vi "MapaIntensidade-FROG.vi"() -> ()   [LabVIEW 2014]
doc: "Mapa de Intensidade FROG\n\nAndré Romero - 2022\nandretec@ifsc.usp.br"
uses:
  FROG-GlobalVar.vi
  <vilib>/Utility/file.llb/Write To Spreadsheet File (DBL).vi
panel:
  in  "stop":bool
  out "Intensity Graph":dbl[][](graph)
  out "Numeric 2":i32
  out "Numeric":i32=4
  out "appended array":dbl[](array[numeric])
  out "Progresso":i32=4
  out "size(s) 2":i32[](array[numeric])=[5, 5]
  out "Array":dbl[][](array[numeric])=[[222.8, 222.8, 222.8, 221.0, 0.0], [220.2, 220.7, 221.6, 222.2, 222.3], [222.4, 222.4, 222.4, 222.5, 0.0], [222.5, 222.5, 222.5, 222.5, 222.5], [0.0, 0.0, 0.0, 0.0, 0.0]]
  out "GO":bool
  out "Temporal FWHM":dbl
  in  "milliseconds to wait":u32=1500
  out "size(s)":i32
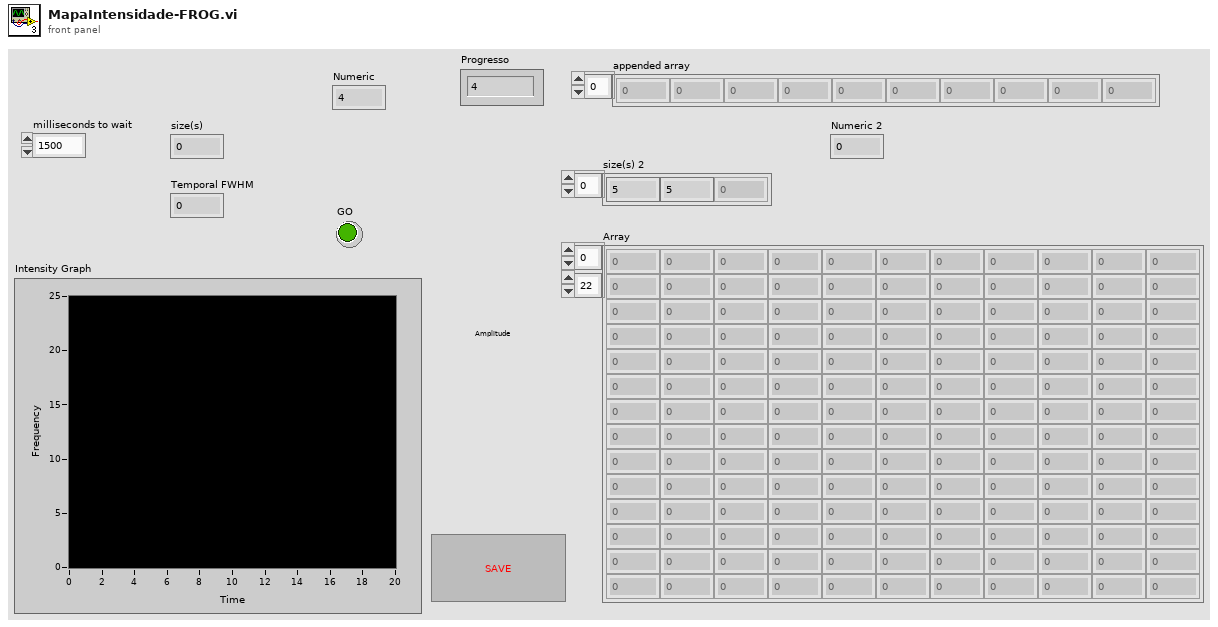
[diagram p1: front panel]
types:
  T1 = typedef "FROG.ctl" = cluster{"Delay increment":dbl, "Center Wavelength":dbl, "Frog Error was":dbl, "Temporal FWHM":dbl, "Spectral FWHM":dbl, "FWHM Time-Bandwidth Product":dbl, "RMS Time-Bandwidth Product":dbl}
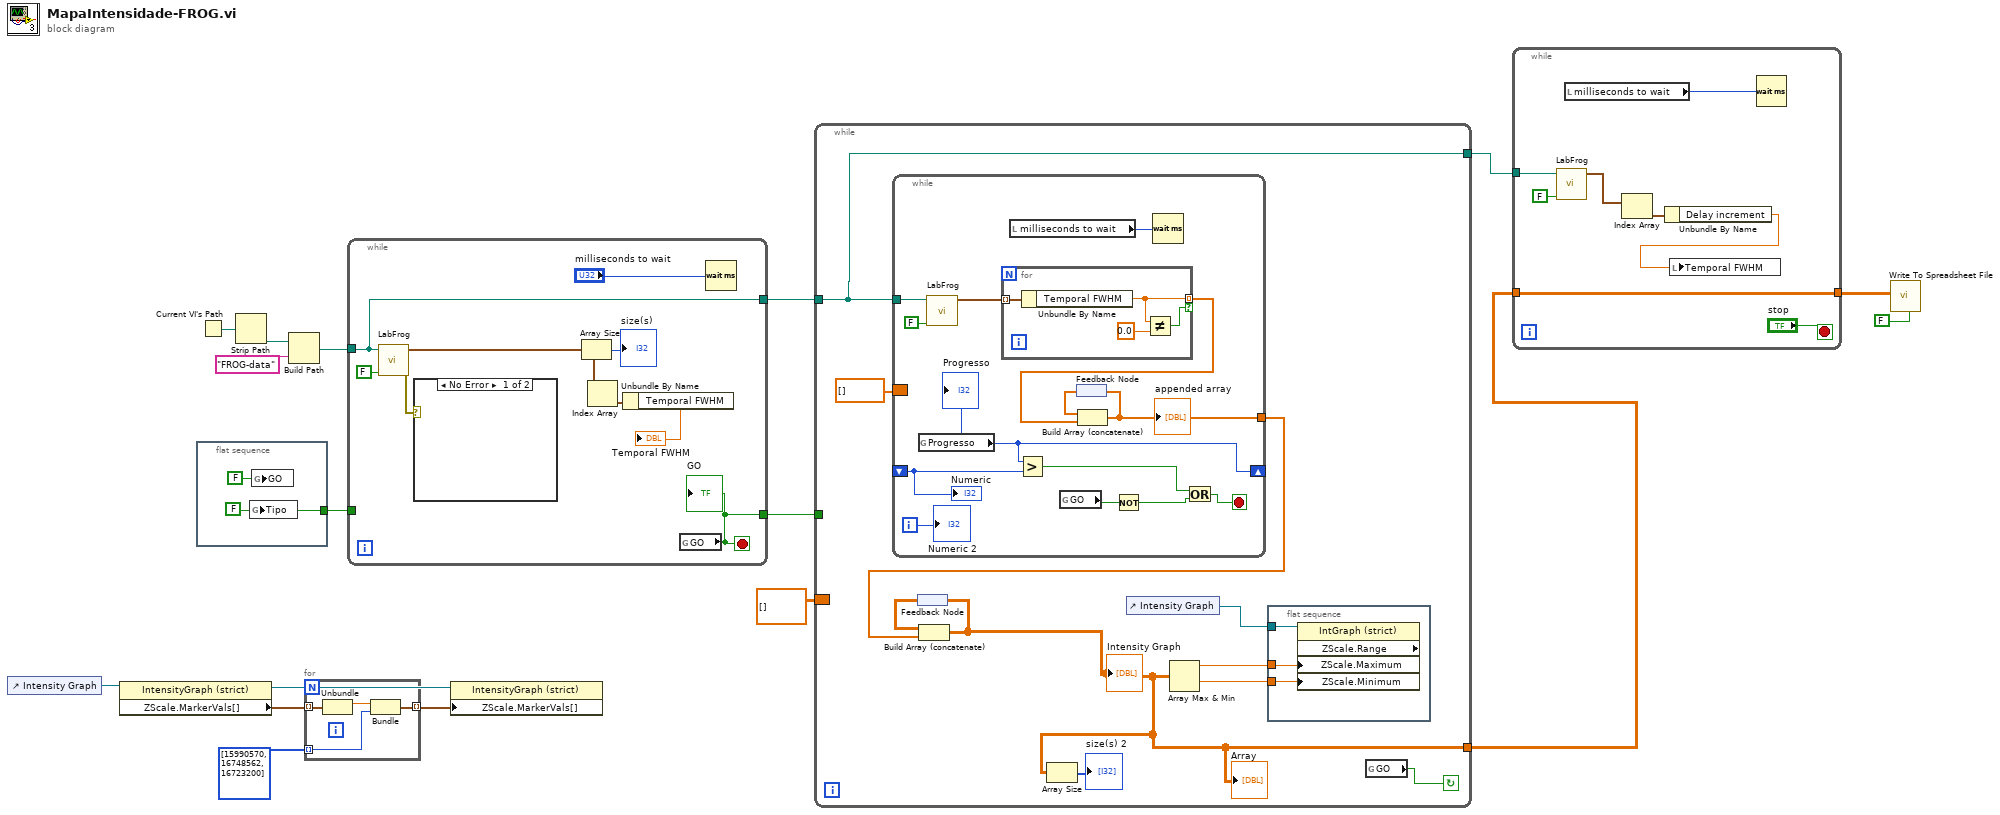
[diagram p0: block diagram]
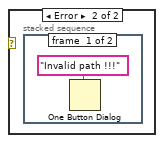
[diagram p2: hidden frame]
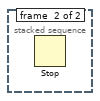
[diagram p3: hidden frame]
diagram:
  n1 = control-ref of="Intensity Graph"() -> (w5:refnum<vi>)
  n2 = property on="Property Node" class="IntensityGraph (strict)"(reference=w5) -> (reference out=w6:refnum<vi>, "ZScale.MarkerVals[]"=w9:cluster{dbl, u32}[])  [unwired: 1 in, 1 out]
  n3 = flat-sequence {
    tunnel: [w18] -> w13
    frame #0 {
      w18 = FALSE ("Tipo")
      n4 = global write "FROG-GlobalVar.vi" "Tipo"(w18) -> ()
      n5 = global write "FROG-GlobalVar.vi" "GO"(FALSE ("GO")) -> ()
    }
  }
  n6 = Current VI's Path() -> (path=w17:path)
  n7 = Strip Path(path=w17) -> (stripped path=w15:path)  [unwired: 1 out]
  n8 = Build Path(base path=w15, name or relative path="FROG-data") -> (appended path=w14:path)
  n9 = for {
    tunnel: w9 -> [w23] mode=indexing
    tunnel: u32[] [15990570, 16748562, 16723200] ("Custom Marker Colors") -> [w21] mode=indexing
    tunnel: [w20] -> w7 mode=indexing
    n10 = Unbundle(w23) -> (w22:dbl)  [unwired: 1 out]
    n11 = Bundle(w22, "Color Box"=w21) -> (w20:cluster{dbl, "Color Box":u32})  [unwired: 1 in]
  }
  n12 = while {
    tunnel: w14 -> [w27]
    tunnel: w13 -> [_]
    tunnel: [w28] -> w12
    tunnel: [w27] -> w11
    stop <- w28 stop-if-true
    n13 = call "LabFrog.vi"("Simutation"=FALSE, "FROG path"=w27) -> ("error out"=w25:errorcluster, "FROG data"=w30:T1[])  [unwired: 8 in]
    n14 = case shown="No Error" w25 {
      frame No Error {
      }
      frame Error {
        n15 = stacked-sequence {
          frame #0 {
            n16 = One Button Dialog(message="Invalid path !!!") -> ()  [unwired: 1 in, 1 out]
          }
          frame #1 {
            n17 = Stop() -> ()  [unwired: 1 in]
          }
        }
      }
    }
    n18 = Array Size(array=w30) -> (size(s)=→"size(s)":i32)
    n19 = Index Array(array=w30) -> (element=w29:T1)  [unwired: 1 in]
    n20 = Unbundle By Name(w29) -> ("Temporal FWHM"=→"Temporal FWHM":dbl)
    n21 = global read "FROG-GlobalVar.vi" "GO"() -> (w28:bool)
    "GO" <- w28
    n22 = Wait (ms)(milliseconds to wait="milliseconds to wait") -> ()  [unwired: 1 out]
  }
  n23 = property on="Property Node" class="IntensityGraph (strict)"(reference=w6, "ZScale.MarkerVals[]"=w7) -> ()  [unwired: 1 in, 2 out]
  n24 = while {
    tunnel: w12 -> [_]
    tunnel: w11 -> [w37]
    border: dbl[][] [] -> [_]
    tunnel: [w37] -> w4
    tunnel: [w34] -> w2
    stop <- w35 continue-if-true
    n25 = while {
      tunnel: w37 -> [w60]
      border: dbl[] [] -> [_]
      shift-right: [w52] -> _
      shift-left: _ -> [w50]
      tunnel: [w53] -> w41
      i -> [w49]
      stop <- w56 stop-if-true
      n26 = global read "FROG-GlobalVar.vi" "Progresso"() -> (w52:i32)
      "Progresso" <- w52
      n27 = call "LabFrog.vi"("Simutation"=FALSE, "FROG path"=w60) -> ("FROG data"=w51:T1[])  [unwired: 8 in, 1 out]
      n28 = for {
        tunnel: w51 -> [w64] mode=indexing
        tunnel: [w61] -> w57 mode=indexing if=w63
        n29 = Unbundle By Name(w64) -> ("Temporal FWHM"=w61:dbl)
        n30 = Not Equal?(x=w61, y=0.0) -> (x != y?=w63:bool)
      }
      n31 = local read "milliseconds to wait"() -> (w59:u32)
      n32 = Greater?(x=w52, y=w50) -> (0:w54:bool)
      n33 = global read "FROG-GlobalVar.vi" "GO"() -> (w55:bool)
      n34 = feedback #1() -> (w58:dbl[])
      n35 = Build Array (concatenate)(w58, w57) -> (w53:dbl[])
      "appended array" <- w53
      n36 = feedback-in #1(w53) -> ()
      n37 = Not(x=w55) -> (.not. x?=w47:bool)
      n38 = Wait (ms)(milliseconds to wait=w59) -> ()  [unwired: 1 out]
      n39 = Or(x=w54, y=w47) -> (x .or. y?=w56:bool)
      "Numeric" <- w50
      "Numeric 2" <- w49
    }
    n40 = feedback #2() -> (w42:dbl[][])
    n41 = Build Array (concatenate)(w42, w41) -> (w34:dbl[][])
    "Intensity Graph" <- w34
    "Array" <- w34
    n42 = feedback-in #2(w34) -> ()
    n43 = Array Size(array=w34) -> (size(s)=→"size(s) 2":i32[])
    n44 = control-ref of="Intensity Graph"() -> (w38:refnum<vi>)
    n45 = Array Max & Min(array=w34) -> (max value=w40:dbl, min value=w39:dbl)  [unwired: 2 out]
    n46 = flat-sequence {
      tunnel: w40 -> [w46]
      tunnel: w39 -> [w45]
      tunnel: w38 -> [w44]
      frame #0 {
        n47 = property on="Property Node" class="IntGraph (strict)" props=["ZScale", "Range", "ZScale", "Maximum", "ZScale", "Minimum"](reference=w44, "ZScale.Maximum"=w46, "ZScale.Minimum"=w45) -> ()  [unwired: 1 in, 3 out]
      }
    }
    n48 = global read "FROG-GlobalVar.vi" "GO"() -> (w35:bool)
  }
  n49 = while {
    tunnel: w4 -> [w72]
    tunnel: w2 -> [w66]
    tunnel: [w66] -> w1
    stop <- "stop" stop-if-true
    n50 = call "LabFrog.vi"("Simutation"=FALSE, "FROG path"=w72) -> ("FROG data"=w70:T1[])  [unwired: 8 in, 1 out]
    n51 = local read "milliseconds to wait"() -> (w65:u32)
    n52 = Index Array(array=w70) -> (element=w69:T1)  [unwired: 1 in]
    n53 = Unbundle By Name(w69) -> ("Delay increment"=w68:dbl)
    n54 = local write "Temporal FWHM"(w68) -> ()
    n55 = Wait (ms)(milliseconds to wait=w65) -> ()  [unwired: 1 out]
  }
  n56 = call-poly <vilib>:"Write To Spreadsheet File.vi"("transpose? (no:F)"=FALSE, "2D data"=w1) -> ()  [unwired: 6 in, 1 out]
